vi "Ctr_FindWithSpecStr.vi"(7 "ClassName(ALL)":string(combo), 8 "error in":errorcluster, 9 "正则表达式(_INC_)":string="_INC_", 11 "vi*(Current VI)":refnum<vi>) -> (0 "error out":errorcluster, 1 "CtrlLables[]":string[](array[string]), 2 "ctrls[]":refnum<vi>[](array[refnum]), 3 "vi* out":refnum<vi>)   [LabVIEW 2016]
uses:
  <vilib>/regexp/Match Regular Expression.xnode
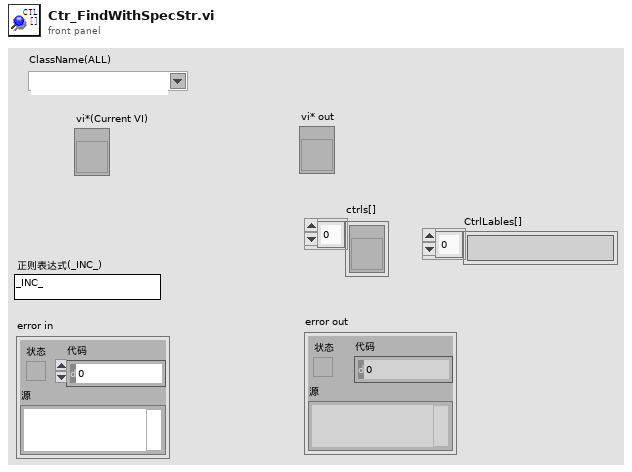
[diagram p1: front panel]
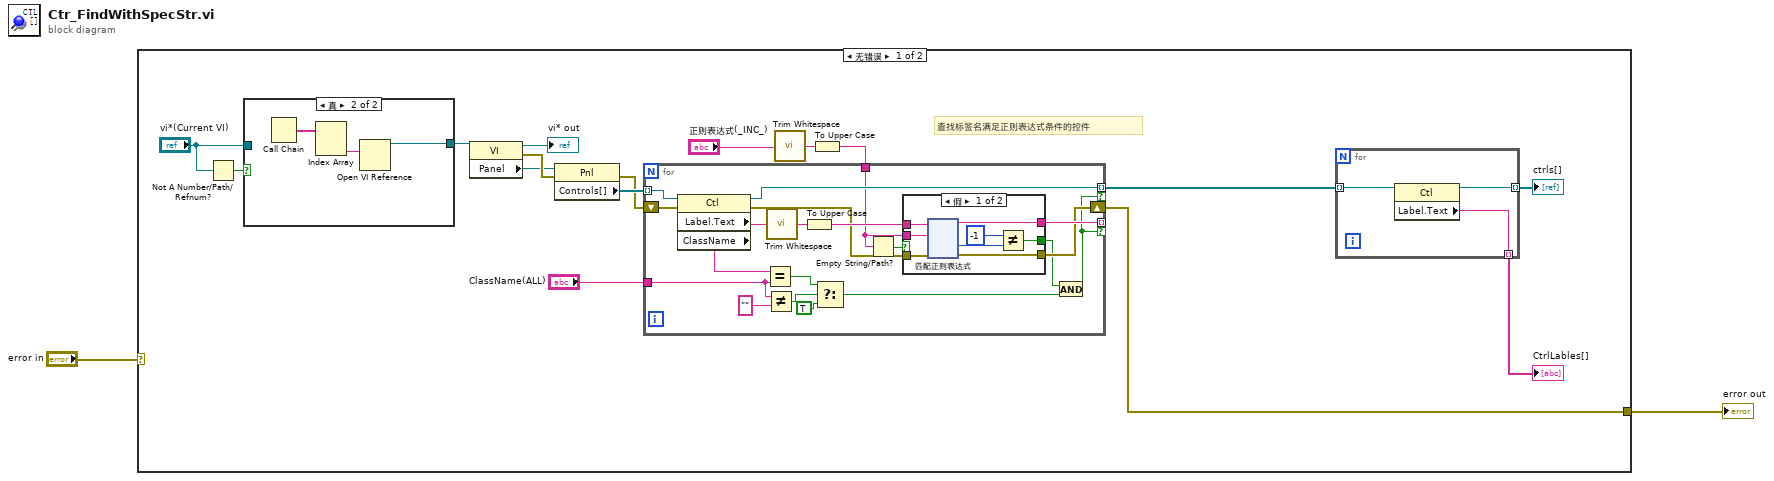
[diagram p0: block diagram]
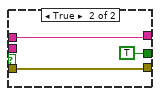
[diagram p3: hidden frame]
diagram:
  n1 = case shown="无错误" "error in" {
    selector: "error in" -> [_ w171]
    tunnel: [w9 w171] -> w1
    frame No Error {
      # "查找标签名满足正则表达式条件的控件"
      n2 = Not A Number/Path/Refnum?(number/path/refnum="vi*(Current VI)") -> (NaN/Path/Refnum?=w13:bool)
      n3 = case shown="真" w13 {
        tunnel: [w22 w25] -> w14
        tunnel: "vi*(Current VI)" -> [w22 _]
        frame False {
        }
        frame True {
          n4 = Call Chain() -> (call chain=w24:string[])
          n5 = Index Array(array=w24) -> (element #2=w23:string)  [unwired: 2 in, 1 out]
          n6 = Open VI Reference(vi path=w23) -> (vi reference=w25:refnum<vi>)  [unwired: 5 in, 1 out]
        }
      }
      n7 = property class="VI"(reference=w14) -> (reference out=→"vi* out":refnum<vi>, error out=w17:errorcluster, "Panel"=w8:refnum<vi>)  [unwired: 1 in]
      n8 = property class="Pnl"(reference=w8, error in=w17) -> (error out=w16:errorcluster, "Controls[]"=w18:refnum<vi>[])  [unwired: 1 out]
      n9 = call <vilib>:"Trim Whitespace.vi"("string"="正则表达式(_INC_)") -> ("trimmed string"=w5:string)  [unwired: 1 in]
      n10 = To Upper Case(1:w5) -> (0:w3:string)
      n11 = for {
        tunnel: w18 -> [w45] mode=indexing
        tunnel: [w44] -> w11 mode=indexing if=w27
        shift-right: [w31] -> w9
        shift-left: w16 -> [w43]
        tunnel: [w33] -> _ mode=indexing if=w27
        tunnel: "ClassName(ALL)" -> [w39]
        tunnel: w3 -> [w30]
        n12 = property class="Ctl"(reference=w45, error in=w43) -> (reference out=w44:refnum<vi>, error out=w32:errorcluster, "Label.Text"=w41:string, "ClassName"=w40:string)
        n13 = Equal?(x=w40, y=w39) -> (x = y?=w36:bool)
        n14 = Not Equal?(x=w39, y="") -> (x != y?=w37:bool)
        n15 = call <vilib>:"Trim Whitespace.vi"("string"=w41) -> ("trimmed string"=w42:string)  [unwired: 1 in]
        n16 = To Upper Case(1:w42) -> (0:w34:string)
        n17 = Select(t=w36, s=w37, f=TRUE) -> (s? t:f=w28:bool)
        n18 = Empty String/Path?(string/path=w30) -> (empty?=w29:bool)
        n19 = case shown="假" w29 {
          tunnel: w34 -> [w53 w170]
          tunnel: [w52 w170] -> w33
          tunnel: w32 -> [w51 w169]
          tunnel: [w50 w169] -> w31
          tunnel: w30 -> [w49 _]
          tunnel: [w46 TRUE] -> w26
          frame False {
            n20 = xnode "匹配正则表达式"("输入字符串"=w53, "正则表达式"=w49, "错误输入"=w51) -> ("匹配之前"=w52:string, "匹配后偏移量"=w48:i32, "错误输出"=w50:errorcluster)  [unwired: 3 in, 2 out]
            n21 = Not Equal?(x=-1, y=w48) -> (x != y?=w46:bool)
          }
          frame True {
          }
        }
        n22 = And(x=w26, y=w28) -> (x .and. y?=w27:bool)
      }
      n23 = for {
        tunnel: w11 -> [w19] mode=indexing
        tunnel: [w21] -> w10 mode=indexing
        tunnel: [w20] -> w6 mode=indexing
        n24 = property class="Ctl"(reference=w19) -> (reference out=w21:refnum<vi>, "Label.Text"=w20:string)  [unwired: 1 in, 1 out]
      }
      "ctrls[]" <- w10
      "CtrlLables[]" <- w6
    }
    frame Error {
    }
  }
  "error out" <- w1
